vi "Validate Measurement Path.vi"(0 "Measurement path":path, 7 "LabVIEW version":string, 11 "error in (no error)":errorcluster) -> (4 "Folder?":bool, 8 "Warning":string, 15 "error out":errorcluster)   [LabVIEW 2021, in "Converter.lvlib"]
uses:
  Converter.lvlib
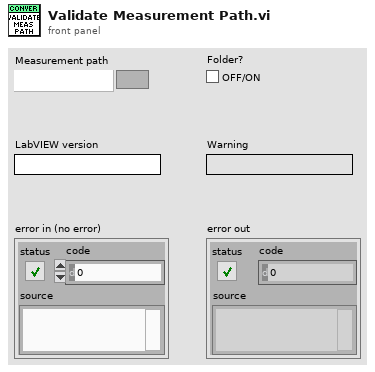
[diagram p1: front panel]
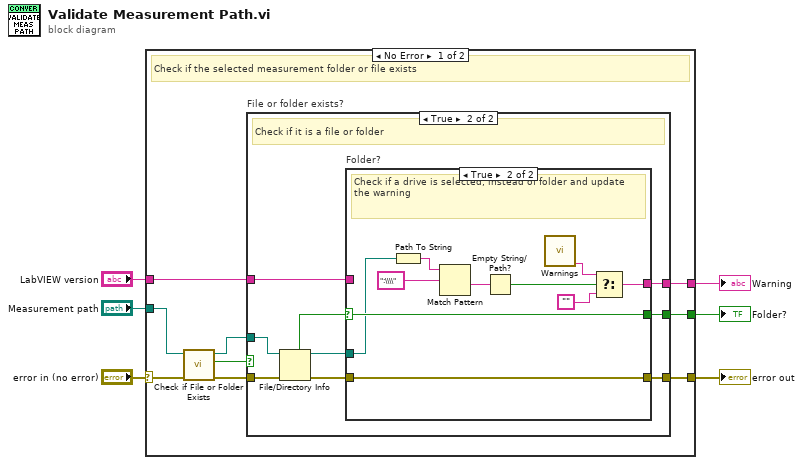
[diagram p0: block diagram]
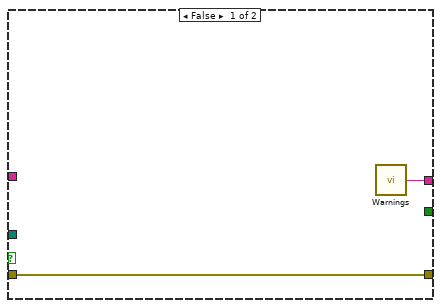
[diagram p2: hidden frame]
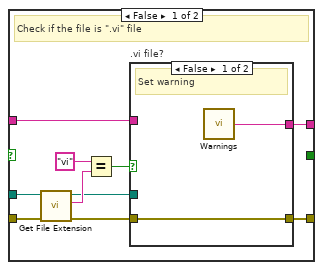
[diagram p3: hidden frame]
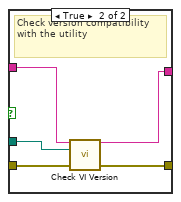
[diagram p4: hidden frame]
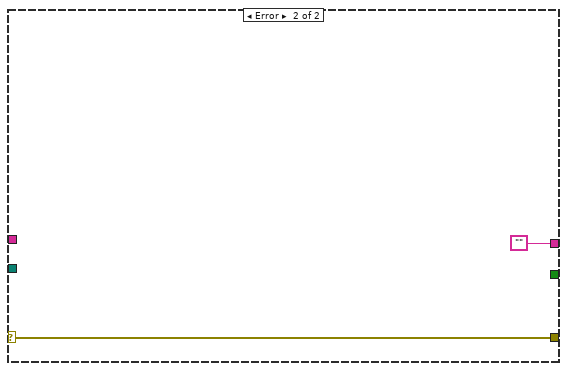
[diagram p5: hidden frame]
diagram:
  n1 = case shown="No Error" "error in (no error)" {
    selector: "error in (no error)" -> [w15 w55]
    tunnel: "Measurement path" -> [w14 _]
    tunnel: [w11 w55] -> w4
    tunnel: [w10 ""] -> w3
    tunnel: "LabVIEW version" -> [w8 _]
    tunnel: [w7 _] -> w1
    frame No Error {
      # "Check if the selected measurement folder or file exists"
      n2 = call <vilib>:"Check if File or Folder Exists.vi"("error in (no error)"=w15, "path"=w14) -> ("error out"=w12:errorcluster, "file or folder exists?"=w13:bool, "dup path"=w9:path)  [unwired: 7 in]
      n3 = case "File or folder exists?" shown="True" w13 {
        tunnel: w12 -> [w16 w25]
        tunnel: [w16 w26] -> w11
        tunnel: [w17 w20] -> w10
        tunnel: w9 -> [_ w22]
        tunnel: w8 -> [_ w19]
        tunnel: [_ w18] -> w7
        frame False {
          n4 = call "Warnings.vi"() -> ("Invalid measurement path"=w17:string)  [unwired: 8 in, 7 out]
        }
        frame True {
          # "Check if it is a file or folder"
          n5 = File/Directory Info(path=w22, error in=w25) -> (path out=w21:path, directory=w23:bool, error out=w24:errorcluster)  [unwired: 4 out]
          n6 = case "Folder?" shown="True" w23 {
            selector: w23 -> [_ w52]
            tunnel: w24 -> [w36 w53]
            tunnel: [w29 w53] -> w26
            tunnel: w21 -> [w35 w46]
            tunnel: [w30 w48] -> w20
            tunnel: w19 -> [w27 _]
            tunnel: [_ w52] -> w18
            frame False {
              # "Check if the file is \".vi\" file"
              n7 = call <vilib>:"Get File Extension.vi"("error in (no error)"=w36, "file"=w35) -> ("error out"=w32:errorcluster, "lowercase file extension"=w34:string, "dup file"=w28:path)  [unwired: 5 in, 2 out]
              n8 = Equal?(x="vi", y=w34) -> (x = y?=w31:bool)
              n9 = case ".vi file?" shown="False" w31 {
                tunnel: w32 -> [w37 w43]
                tunnel: [w38 w41] -> w30
                tunnel: [w37 w40] -> w29
                tunnel: w28 -> [_ w39]
                tunnel: w27 -> [_ w42]
                frame False {
                  # "Set warning"
                  n10 = call "Warnings.vi"() -> ("Invalid measurement path"=w38:string)  [unwired: 8 in, 7 out]
                }
                frame True {
                  # "Check version compatibility with the utility"
                  n11 = call "Check VI Version.vi"("LabVIEW version"=w42, "VI path"=w39, "error in (no error)"=w43) -> ("Incompatible version warning"=w41:string, "error out"=w40:errorcluster)  [unwired: 11 in]
                }
              }
            }
            frame True {
              # "Check if a drive is selected, instead of folder and update the warning"
              n12 = Path To String(path=w46) -> (string=w45:string)
              n13 = Match Pattern(string=w45, regular expression=":\\\\") -> (after substring=w51:string)  [unwired: 1 in, 3 out]
              n14 = Empty String/Path?(string/path=w51) -> (empty?=w44:bool)
              n15 = call "Warnings.vi"() -> ("Drive selection"=w47:string)  [unwired: 8 in, 7 out]
              n16 = Select(t=w47, s=w44, f="") -> (s? t:f=w48:string)
            }
          }
        }
      }
    }
    frame Error {
    }
  }
  "error out" <- w4
  "Warning" <- w3
  "Folder?" <- w1
